vi "SetSensorWidth.vi"(8 "error in (no error)":errorcluster, 10 "Sensor.SensorWidth(Pixel)":i32, 11 "Camera in":refnum<class "Camera.lvclass">) -> (0 "error out":errorcluster, 3 "Camera out":refnum<class "Camera.lvclass">)   [LabVIEW 2020, in "Camera.lvlib" / "Camera.lvclass"]
uses:
  Camera.lvclass
  Camera.lvclass/Camera.ctl
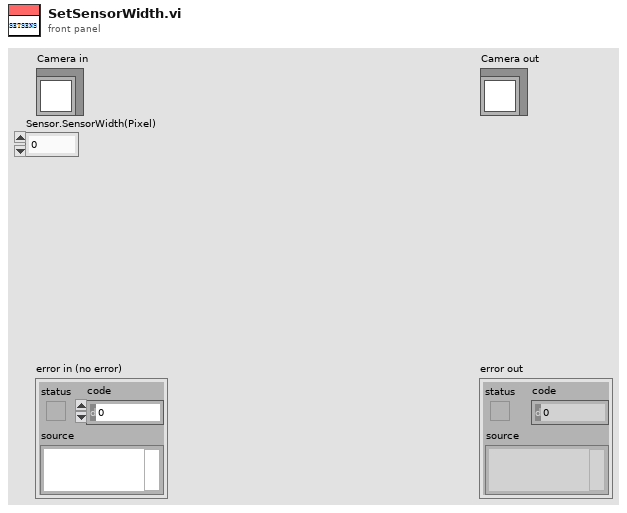
[diagram p1: front panel]
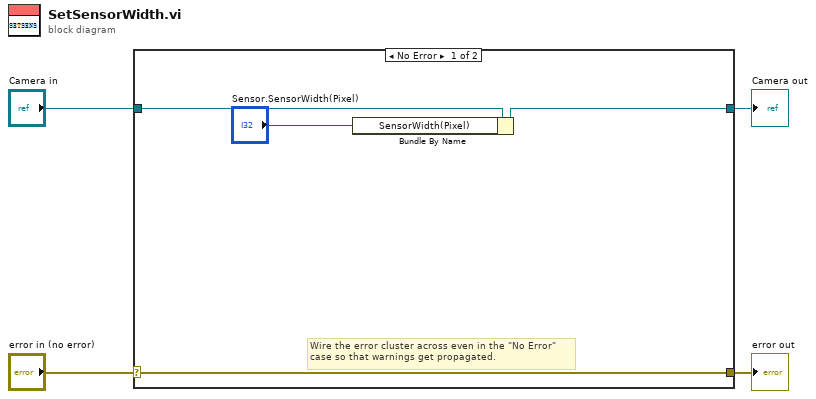
[diagram p0: block diagram]
diagram:
  n1 = case shown="No Error" "error in (no error)" {
    selector: "error in (no error)" -> [w7 w10]
    tunnel: [w7 w10] -> w3
    tunnel: [w6 w9] -> w1
    tunnel: "Camera in" -> [w8 w9]
    frame No Error {
      # "Wire the error cluster across even in the \"No Error\"\ncase so that warnings get propagated."
      n2 = Bundle By Name(cluster=w8, "SensorWidth(Pixel)"="Sensor.SensorWidth(Pixel)") -> (w6:refnum<class "Camera.lvclass">)
    }
    frame Error {
    }
  }
  "error out" <- w3
  "Camera out" <- w1
